vi "BO_initvi.vi"(8 "출력 클러스터 2":T1, 9 "Stride number":u32, 10 "Initialize":bool, 11 "R_NUM":u32) -> (0 "출력 클러스터 3":T1)   [LabVIEW 2019]
uses:
  <vilib>/numeric/Random Number (Range) I64.vi
  <vilib>/numeric/sub_Random U32.vi
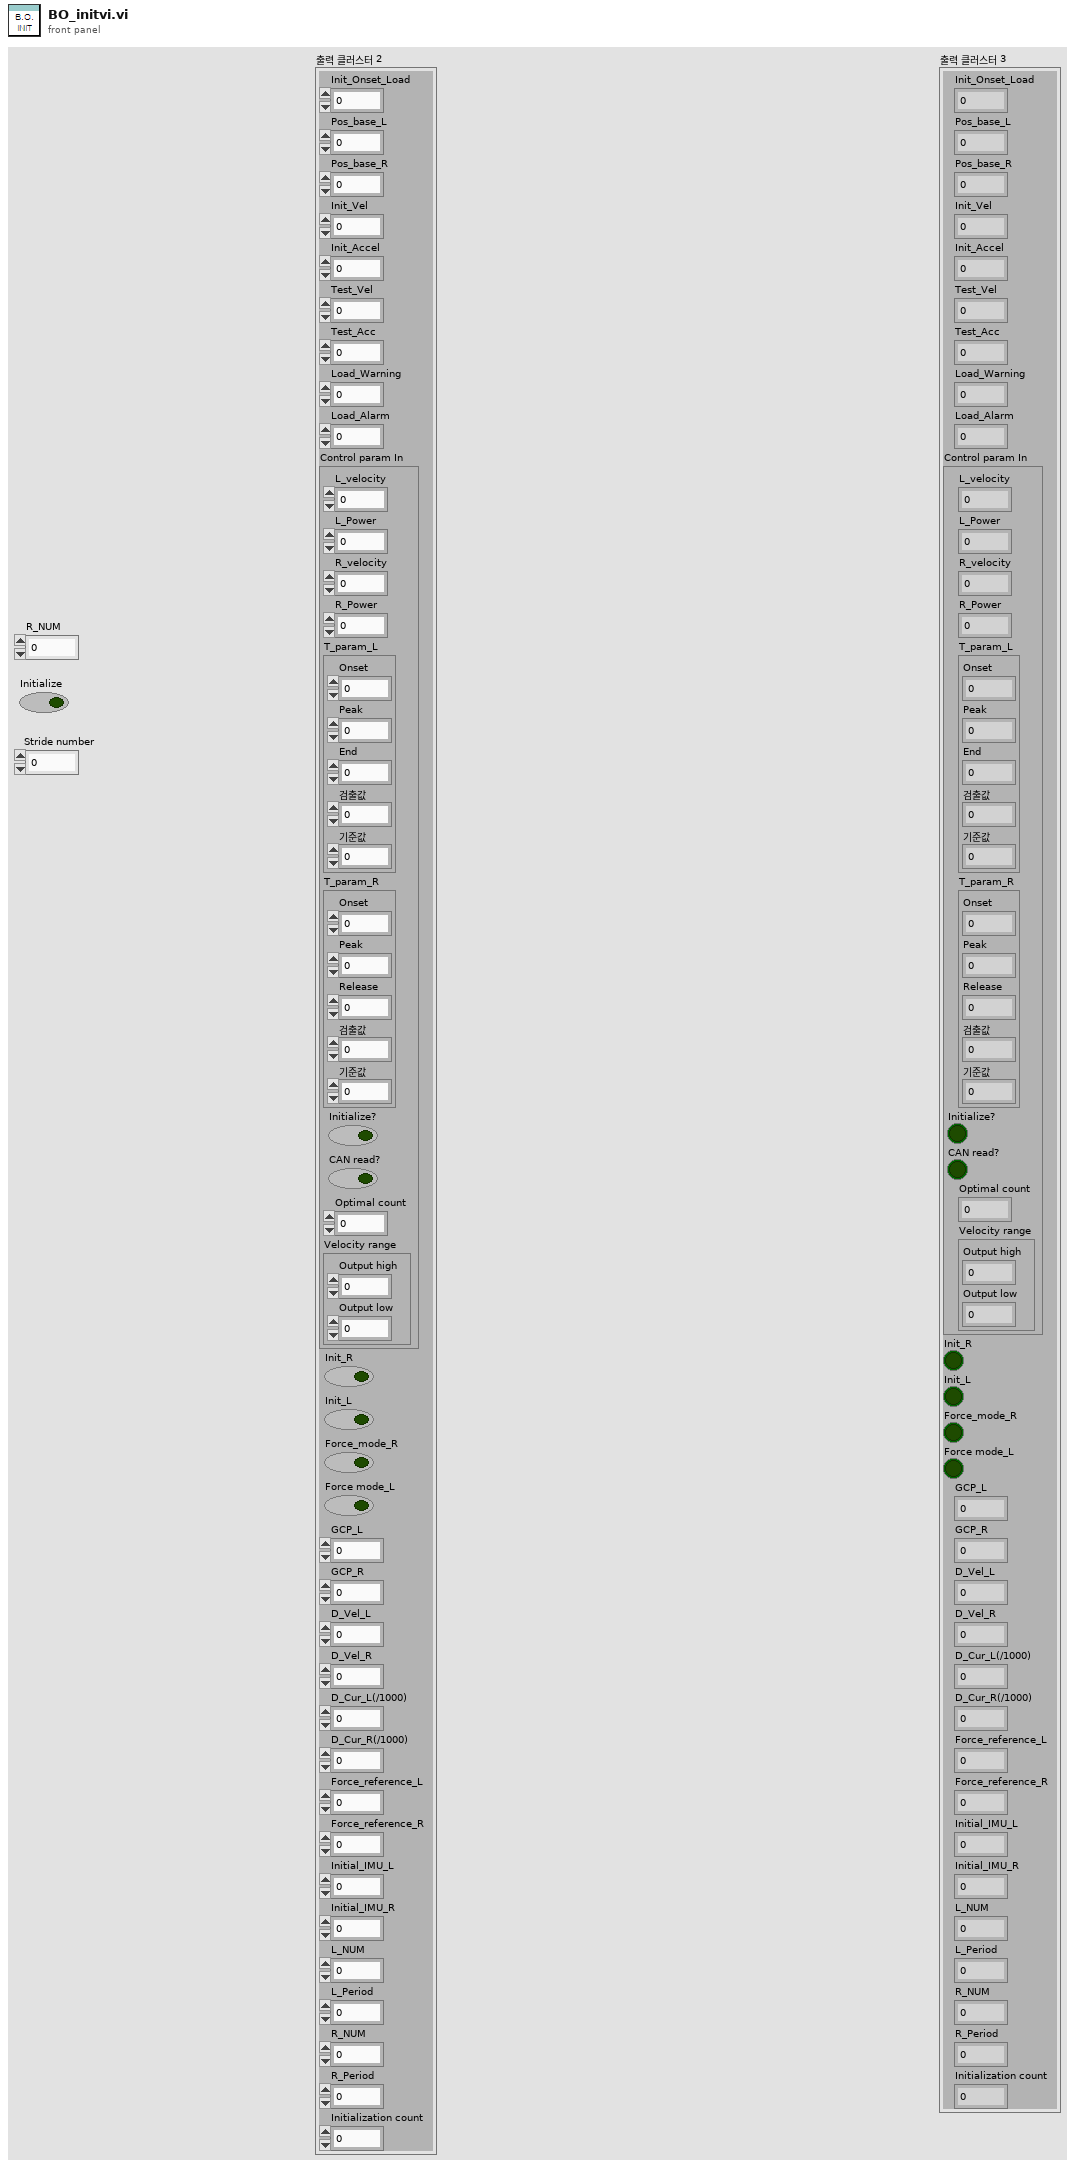
[diagram p1: front panel]
types:
  T1 = cluster{"Init_Onset_Load":sgl, "Pos_base_L":sgl, "Pos_base_R":sgl, "Init_Vel":i32, "Init_Accel":u32, "Test_Vel":i32, "Test_Acc":u32, "Load_Warning":sgl, "Load_Alarm":sgl, "Control param In":cluster{"L_velocity":u32, "L_Power":sgl, "R_velocity":u32, "R_Power":sgl, "T_param_L":cluster{"Onset":sgl, "Peak":sgl, "End":sgl, "검출값":sgl, "기준값":sgl}, "T_param_R":cluster{"Onset":sgl, "Peak":sgl, "Release":sgl, "검출값":sgl, "기준값":sgl}, "Initialize?":bool, "CAN read?":bool, "Optimal count":i32, "Velocity range":cluster{"Output high":dbl, "Output low":dbl}}, "Init_R":bool, "Init_L":bool, "Force_mode_R":bool, "Force mode_L":bool, "GCP_L":sgl, "GCP_R":sgl, "D_Vel_L":sgl, "D_Vel_R":sgl, "D_Cur_L(/1000)":sgl, "D_Cur_R(/1000)":sgl, "Force_reference_L":sgl, "Force_reference_R":sgl, "Initial_IMU_L":sgl, "Initial_IMU_R":sgl, "L_NUM":u32, "L_Period":i16, "R_NUM":u32, "R_Period":i16, "Initialization count":i32}
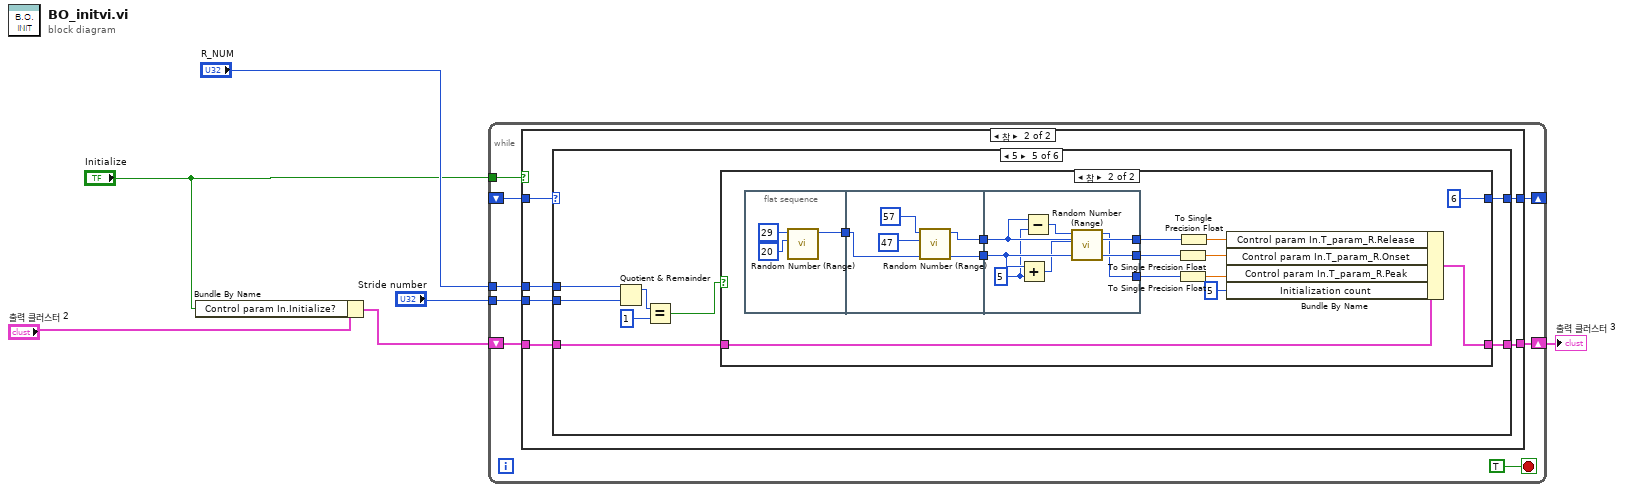
[diagram p0: block diagram]
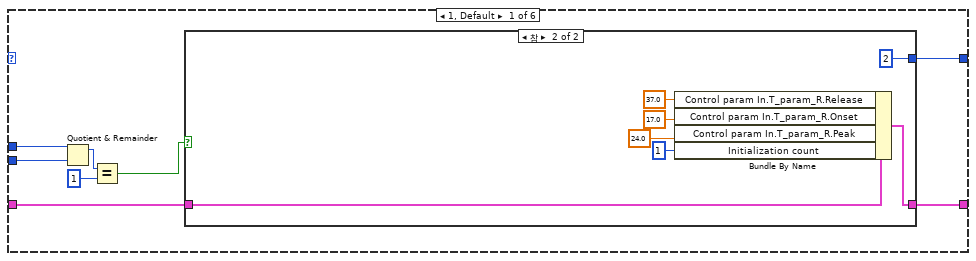
[diagram p3: hidden frame]
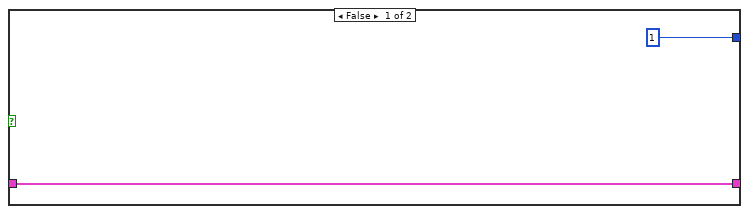
[diagram p4: hidden frame]
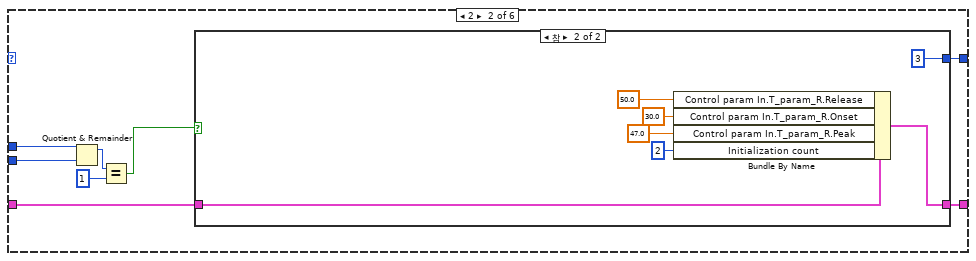
[diagram p5: hidden frame]
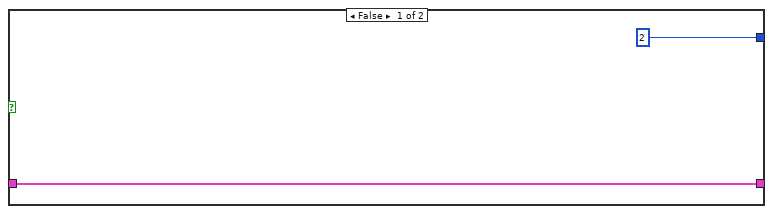
[diagram p6: hidden frame]
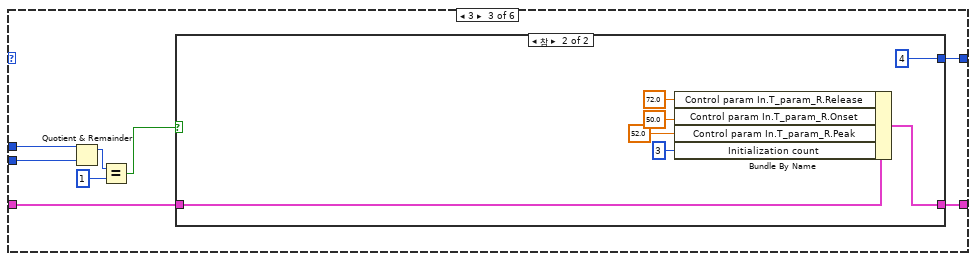
[diagram p7: hidden frame]
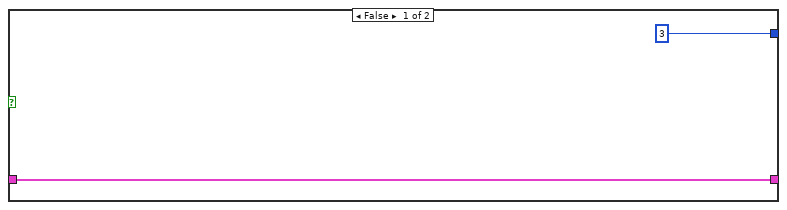
[diagram p8: hidden frame]
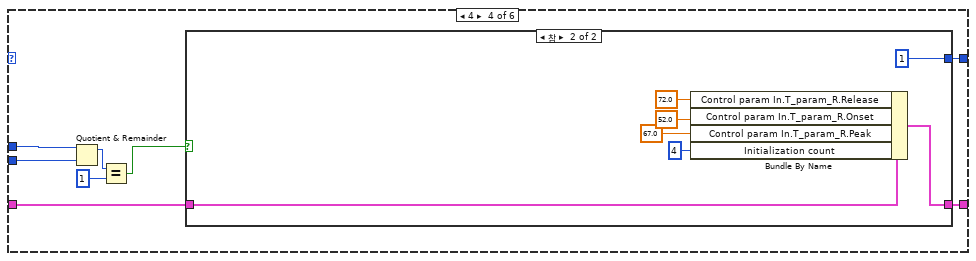
[diagram p9: hidden frame]
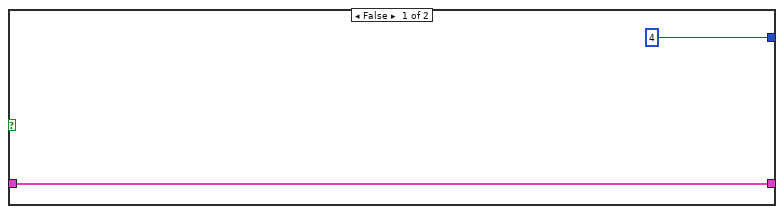
[diagram p10: hidden frame]
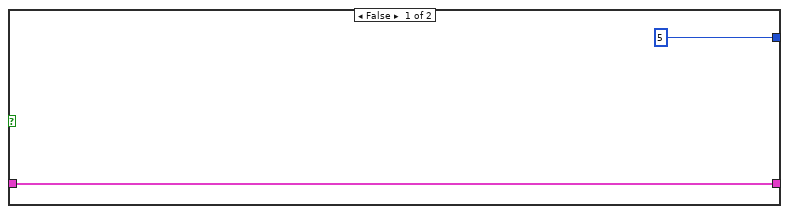
[diagram p11: hidden frame]
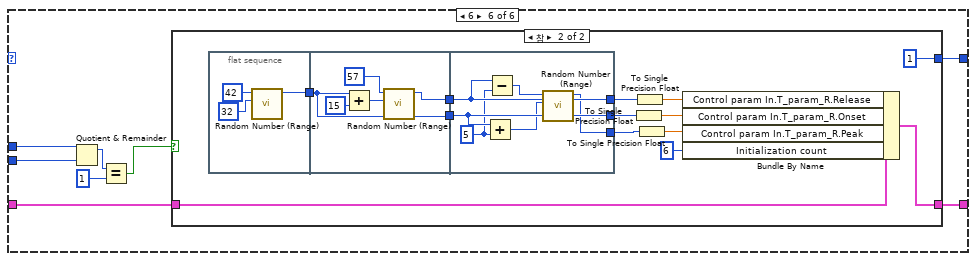
[diagram p12: hidden frame]
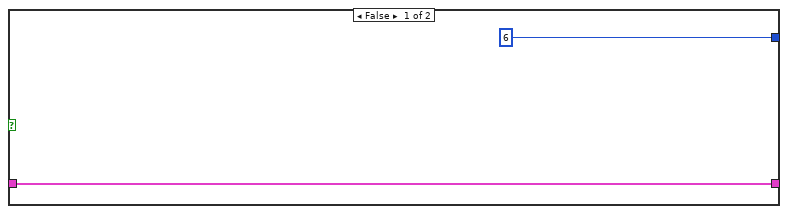
[diagram p13: hidden frame]
diagram:
  n1 = Bundle By Name(cluster="출력 클러스터 2", "Control param In.Initialize?"="Initialize") -> (w3:T1)
  n2 = while {
    tunnel: "R_NUM" -> [w13]
    tunnel: "Initialize" -> [w11]
    shift-right: [w14] -> w1
    shift-left: w3 -> [w12]
    shift-right: [w9] -> _
    shift-left: _ -> [w8]
    tunnel: "Stride number" -> [w7]
    stop <- TRUE stop-if-true
    n3 = case shown="참" w11 {
      tunnel: w13 -> [_ w20]
      tunnel: w12 -> [w16 w22]
      tunnel: [w16 w21] -> w14
      tunnel: [w15 w19] -> w9
      tunnel: w8 -> [w15 w18]
      tunnel: w7 -> [_ w17]
      frame False {
      }
      frame True {
        n4 = case shown="5" w18 {
          tunnel: w22 -> [w30 w47 w64 w81 w98 w134]
          tunnel: [w29 w46 w63 w80 w97 w133] -> w21
          tunnel: w20 -> [w25 w42 w59 w76 w93 w129]
          tunnel: [w26 w43 w60 w77 w94 w130] -> w19
          tunnel: w17 -> [w24 w41 w58 w75 w92 w128]
          frame 1, Default {
            n5 = Quotient & Remainder(x=w25, y=w24) -> (x-y*floor(x/y)=w28:u32)  [unwired: 1 out]
            n6 = Equal?(x=w28, y=u32 1) -> (x = y?=w23:bool)
            n7 = case shown="참" w23 {
              tunnel: w30 -> [w32 w38]
              tunnel: [w32 w39] -> w29
              tunnel: [1 2] -> w26
              frame False {
              }
              frame True {
                n8 = Bundle By Name(cluster=w38, "Control param In.T_param_R.Release"=sgl 37.0, "Control param In.T_param_R.Onset"=sgl 17.0, "Control param In.T_param_R.Peak"=sgl 24.0, "Initialization count"=1) -> (w39:T1)
              }
            }
          }
          frame 2 {
            n9 = Quotient & Remainder(x=w42, y=w41) -> (x-y*floor(x/y)=w45:u32)  [unwired: 1 out]
            n10 = Equal?(x=w45, y=u32 1) -> (x = y?=w40:bool)
            n11 = case shown="참" w40 {
              tunnel: w47 -> [w49 w55]
              tunnel: [w49 w56] -> w46
              tunnel: [2 3] -> w43
              frame False {
              }
              frame True {
                n12 = Bundle By Name(cluster=w55, "Control param In.T_param_R.Release"=sgl 50.0, "Control param In.T_param_R.Onset"=sgl 30.0, "Control param In.T_param_R.Peak"=sgl 47.0, "Initialization count"=2) -> (w56:T1)
              }
            }
          }
          frame 3 {
            n13 = Quotient & Remainder(x=w59, y=w58) -> (x-y*floor(x/y)=w62:u32)  [unwired: 1 out]
            n14 = Equal?(x=w62, y=u32 1) -> (x = y?=w57:bool)
            n15 = case shown="참" w57 {
              tunnel: w64 -> [w66 w72]
              tunnel: [w66 w73] -> w63
              tunnel: [3 4] -> w60
              frame False {
              }
              frame True {
                n16 = Bundle By Name(cluster=w72, "Control param In.T_param_R.Release"=sgl 72.0, "Control param In.T_param_R.Onset"=sgl 50.0, "Control param In.T_param_R.Peak"=sgl 52.0, "Initialization count"=3) -> (w73:T1)
              }
            }
          }
          frame 4 {
            n17 = Quotient & Remainder(x=w76, y=w75) -> (x-y*floor(x/y)=w79:u32)  [unwired: 1 out]
            n18 = Equal?(x=w79, y=u32 1) -> (x = y?=w74:bool)
            n19 = case shown="참" w74 {
              tunnel: w81 -> [w83 w89]
              tunnel: [w83 w90] -> w80
              tunnel: [4 1] -> w77
              frame False {
              }
              frame True {
                n20 = Bundle By Name(cluster=w89, "Control param In.T_param_R.Release"=sgl 72.0, "Control param In.T_param_R.Onset"=sgl 52.0, "Control param In.T_param_R.Peak"=sgl 67.0, "Initialization count"=4) -> (w90:T1)
              }
            }
          }
          frame 5 {
            n21 = Quotient & Remainder(x=w93, y=w92) -> (x-y*floor(x/y)=w96:u32)  [unwired: 1 out]
            n22 = Equal?(x=w96, y=u32 1) -> (x = y?=w91:bool)
            n23 = case shown="참" w91 {
              tunnel: w98 -> [w100 w110]
              tunnel: [w100 w113] -> w97
              tunnel: [5 6] -> w94
              frame False {
              }
              frame True {
                n24 = flat-sequence {
                  tunnel: [w114] -> w109
                  tunnel: w109 -> [w118]
                  tunnel: [w119] -> w105
                  tunnel: [w118] -> w104
                  tunnel: [w126] -> w107
                  tunnel: [w124] -> w108
                  tunnel: w105 -> [w124]
                  tunnel: w104 -> [w126]
                  tunnel: [w121] -> w102
                  frame #0 {
                    n25 = call-poly <vilib>:"Random Number (Range).vi"("lower bound (-100)"=i64 20 ("lower bound (0)"), "upper bound (100)"=i64 29) -> ("number"=w114:i64)  [unwired: 9 in]
                  }
                  frame #1 {
                    n26 = call-poly <vilib>:"Random Number (Range).vi"("lower bound (-100)"=i64 47 ("x"), "upper bound (100)"=i64 57) -> ("number"=w119:i64)  [unwired: 9 in]
                  }
                  frame #2 {
                    w123 = i64 5 ("y")
                    n27 = Add(x=w126, y=w123) -> (x+y=w125:i64)
                    n28 = Subtract(x=w124, y=w123) -> (x-y=w122:i64)
                    n29 = call-poly <vilib>:"Random Number (Range).vi"("lower bound (-100)"=w125, "upper bound (100)"=w122) -> ("number"=w121:i64)  [unwired: 9 in]
                  }
                }
                n30 = To Single Precision Float(number=w107) -> (single precision float=w111:sgl)
                n31 = To Single Precision Float(number=w102) -> (single precision float=w103:sgl)
                n32 = To Single Precision Float(number=w108) -> (single precision float=w112:sgl)
                n33 = Bundle By Name(cluster=w110, "Control param In.T_param_R.Release"=w112, "Control param In.T_param_R.Onset"=w111, "Control param In.T_param_R.Peak"=w103, "Initialization count"=5) -> (w113:T1)
              }
            }
          }
          frame 6 {
            n34 = Quotient & Remainder(x=w129, y=w128) -> (x-y*floor(x/y)=w132:u32)  [unwired: 1 out]
            n35 = Equal?(x=w132, y=u32 1) -> (x = y?=w127:bool)
            n36 = case shown="참" w127 {
              tunnel: w134 -> [w136 w146]
              tunnel: [w136 w149] -> w133
              tunnel: [6 1] -> w130
              frame False {
              }
              frame True {
                n37 = flat-sequence {
                  tunnel: [w150] -> w145
                  tunnel: w145 -> [w153]
                  tunnel: [w154] -> w141
                  tunnel: [w153] -> w140
                  tunnel: [w163] -> w143
                  tunnel: [w162] -> w144
                  tunnel: w141 -> [w162]
                  tunnel: w140 -> [w163]
                  tunnel: [w158] -> w139
                  frame #0 {
                    n38 = call-poly <vilib>:"Random Number (Range).vi"("lower bound (-100)"=i64 32 ("lower bound (0)"), "upper bound (100)"=i64 42) -> ("number"=w150:i64)  [unwired: 9 in]
                  }
                  frame #1 {
                    n39 = Add(x=w153, y=i64 15 ("x")) -> (x+y=w157:i64)
                    n40 = call-poly <vilib>:"Random Number (Range).vi"("lower bound (-100)"=w157, "upper bound (100)"=i64 57) -> ("number"=w154:i64)  [unwired: 9 in]
                  }
                  frame #2 {
                    w161 = i64 5 ("y")
                    n41 = Add(x=w163, y=w161) -> (x+y=w159:i64)
                    n42 = Subtract(x=w162, y=w161) -> (x-y=w160:i64)
                    n43 = call-poly <vilib>:"Random Number (Range).vi"("lower bound (-100)"=w159, "upper bound (100)"=w160) -> ("number"=w158:i64)  [unwired: 9 in]
                  }
                }
                n44 = To Single Precision Float(number=w143) -> (single precision float=w147:sgl)
                n45 = To Single Precision Float(number=w144) -> (single precision float=w148:sgl)
                n46 = To Single Precision Float(number=w139) -> (single precision float=w138:sgl)
                n47 = Bundle By Name(cluster=w146, "Control param In.T_param_R.Release"=w148, "Control param In.T_param_R.Onset"=w147, "Control param In.T_param_R.Peak"=w138, "Initialization count"=6) -> (w149:T1)
              }
            }
          }
        }
      }
    }
  }
  "출력 클러스터 3" <- w1
